vi "Sync.Destroy.vi"(8 "error in (no error)":errorcluster, 11 "DAQmx in":refnum<class "DAQmx.lvclass">) -> (0 "error out":errorcluster, 3 "DAQmx out":refnum<class "DAQmx.lvclass">)   [LabVIEW 2019, in "DAQmx.lvclass"]
uses:
  DAQmx.lvclass
  DAQmx.lvclass/DAQmx.ctl
  typedefs/DAQmx.Channel Map--Cluster.ctl
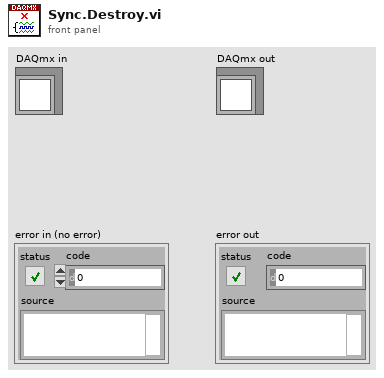
[diagram p1: front panel]
types:
  T1 = typedef "DAQmx.lvclass/DAQmx.Channel Map--Cluster.ctl" = cluster{"task":refnum<k21>, "Device":tag, "Offset":u32, "Count":u32}
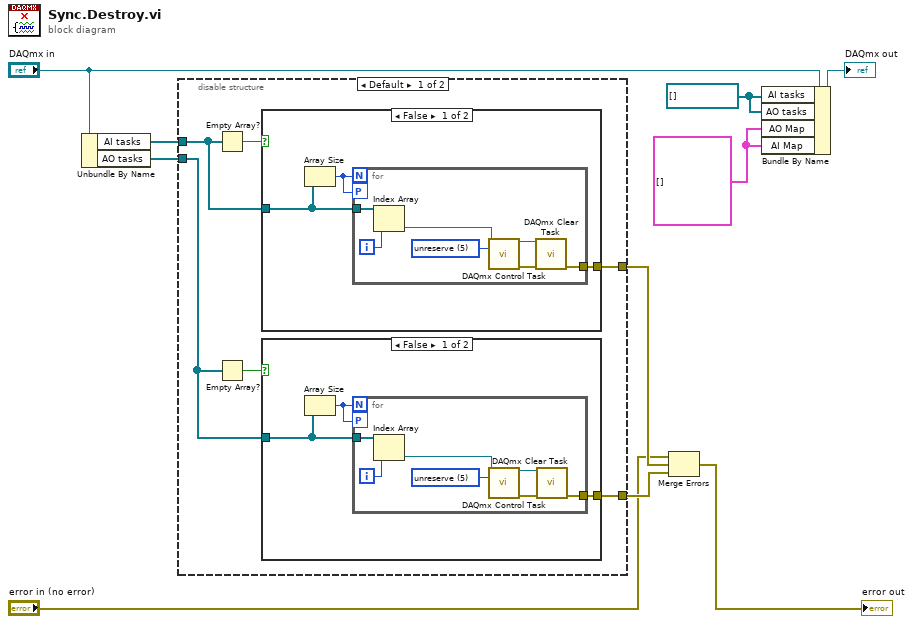
[diagram p0: block diagram]
diagram:
  w1 = T1[] [] ("AO Map")
  w2 = refnum<k21>[] [] ("AI task")
  n1 = Unbundle By Name("DAQmx in") -> ("AI tasks"=w9:refnum<k21>[], "AO tasks"=w10:refnum<k21>[])
  n2 = disable-structure shown="Default" {
    disable-tunnel: [w16 _] -> w5
    disable-tunnel: w10 -> [w13 _]
    disable-tunnel: w9 -> [w14 _]
    disable-tunnel: [w12 _] -> w6
    frame condition #0 (active) {
      n3 = Empty Array?(array=w14) -> (empty?=w15:bool)
      n4 = Empty Array?(array=w13) -> (empty?=w11:bool)
      n5 = case shown="False" w15 {
        tunnel: w14 -> [w28 _]
        tunnel: [w29 _] -> w16
        frame False {
          n6 = Array Size(array=w28) -> (size(s)=w27:i32)
          n7 = for {
            N: w27 -> [_]
            tunnel: w28 -> [w35]
            tunnel: [w31] -> w29
            workers-P: w27 -> [_]
            i -> [w36]
            w34 = 5 items=["verify"=2, "reserve"=4, "commit"=3, "unreserve"=5, "abort"=6] ("action")
            n8 = Index Array(array=w35, index=w36) -> (element=w33:refnum<k21>)
            n9 = call <vilib>:"DAQmx Control Task.vi"("task/channels in"=w33, "action"=w34) -> ("task out"=w30:refnum<k21>, "error out"=w32:errorcluster)  [unwired: 12 in]
            n10 = call <vilib>:"DAQmx Clear Task.vi"("task in"=w30, "error in"=w32) -> ("error out"=w31:errorcluster)  [unwired: 13 in]
          }
        }
        frame True {
        }
      }
      n11 = case shown="False" w11 {
        tunnel: w13 -> [w18 _]
        tunnel: [w19 _] -> w12
        frame False {
          n12 = Array Size(array=w18) -> (size(s)=w17:i32)
          n13 = for {
            N: w17 -> [_]
            tunnel: w18 -> [w25]
            tunnel: [w20] -> w19
            workers-P: w17 -> [_]
            i -> [w26]
            w24 = 5 items=["verify"=2, "reserve"=4, "commit"=3, "unreserve"=5, "abort"=6] ("action")
            n14 = Index Array(array=w25, index=w26) -> (element=w23:refnum<k21>)
            n15 = call <vilib>:"DAQmx Control Task.vi"("task/channels in"=w23, "action"=w24) -> ("task out"=w22:refnum<k21>, "error out"=w21:errorcluster)  [unwired: 12 in]
            n16 = call <vilib>:"DAQmx Clear Task.vi"("task in"=w22, "error in"=w21) -> ("error out"=w20:errorcluster)  [unwired: 13 in]
          }
        }
        frame True {
        }
      }
    }
    frame condition #1 {
    }
  }
  n17 = Merge Errors("error in (no error)", w5, w6) -> (→"error out":errorcluster)
  n18 = Bundle By Name(cluster="DAQmx in", "AI tasks"=w2, "AO tasks"=w2, "AO Map"=w1, "AI Map"=w1) -> (→"DAQmx out":refnum<class "DAQmx.lvclass">)
